vi "Sensors Get.vi"   [LabVIEW 2013]
uses:
  Sensors Global Data.vi
types:
  T1 = typedef "WPI_GyroDevRef.ctl" = cluster{"DevStatus":errorcluster, "Analog Module":T2, "Analog Channel":T3, "Offset":dbl, "Gain (VoltsPerDegree/Second)":dbl}
  T2 = typedef "FPGA_TypedefAnalogModule.ctl" = enum16{"Analog Module 1", "Analog Module 2"}
  T3 = typedef "FPGA_AIChannel.ctl" = enum8{"AI 1", "AI 2", "AI 3", "AI 4", "AI 5", "AI 6", "AI 7", "AI 8", "Invalid"}
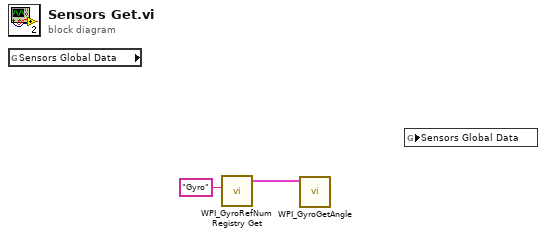
[diagram p0: block diagram]
diagram:
  n1 = global read "Sensors Global Data.vi" "Sensors Global Data"() -> ()  [unwired: 1 out]
  n2 = call <vilib>:"WPI_GyroRefNum Registry Get.vi"("refnum name"="Gyro") -> ("GyroDevRef"=w2:T1)  [unwired: 9 in, 1 out]
  n3 = call <vilib>:"WPI_GyroGetAngle.vi"("GyroDevRef"=w2) -> ()  [unwired: 7 in, 4 out]
  n4 = global read "Sensors Global Data.vi" "Sensors Global Data"() -> ()  [unwired: 1 in]
